vi "Filename - Is Class.vi"(1 "Filename (including file extension)":string) -> (0 "Is Class?":bool)   [LabVIEW 2021]
doc: "Returns True if the input Filename is that of a Class"
panel:
  # "Development\ncontrols/indicators useful for development and testing, but which are not outputs of the VI"
  # "Input\nInputs to the VI"
  # "Output\nOutputs of the VI"
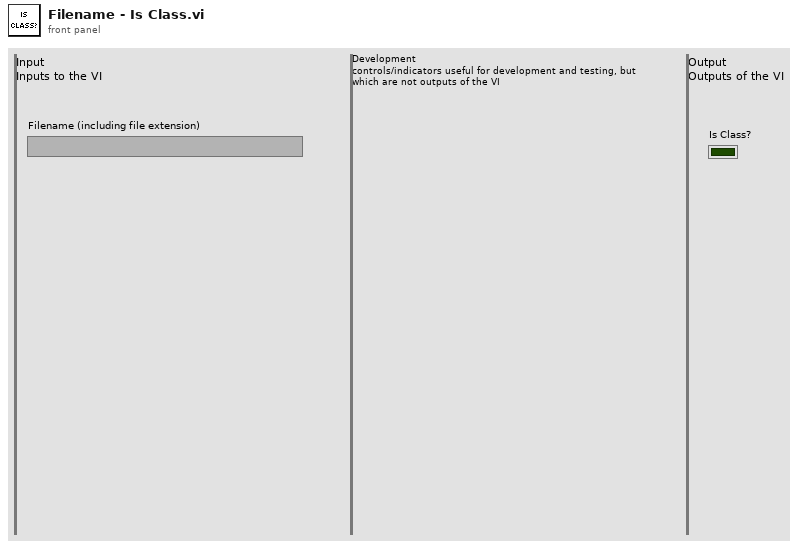
[diagram p1: front panel]
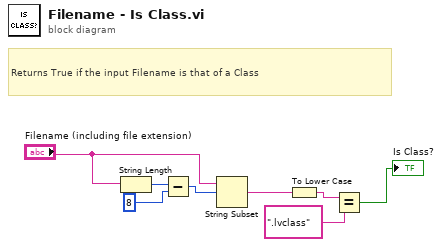
[diagram p0: block diagram]
diagram:
  # "Returns True if the input Filename is that of a Class"
  n1 = String Length(string="Filename (including file extension)") -> (length=w6:i32)
  n2 = Subtract(x=w6, y=8) -> (x-y=w7:i32)
  n3 = String Subset(string="Filename (including file extension)", offset (0)=w7) -> (substring=w8:string)  [unwired: 1 in]
  n4 = To Lower Case(string=w8) -> (all lower case string=w3:string)
  n5 = Equal?(x=w3, y=".lvclass") -> (x = y?=→"Is Class?":bool)
